vi "Write_Current_Row_to_log_file.vi"(0 "Current Time":dbl, 1 "Channel Names":string[](array[string]), 2 "Channel Values":string[](array[string]), 3 "Comments":string[](array[string]), 4 "User added comment":string) -> (7 "File Updated?":bool)   [LabVIEW 2020]
uses:
  ADAM_Global.vi
  Anemometry/Anemometry Sub Vis/Globals/Preference_global.vi
  Anemometry/Anemometry Sub Vis/Globals/Constants_global.vi
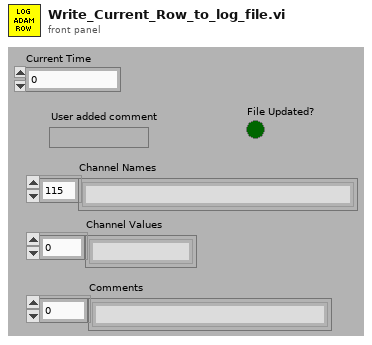
[diagram p1: front panel]
types:
  T1 = typedef "LVDateTimeRec.ctl" = cluster{"fractional second":dbl, "second":i32, "minute":i32, "hour":i32, "day of month":i32, "month":i32, "year":i32, "day of week":i32, "day of year":i32, "DST":i32}
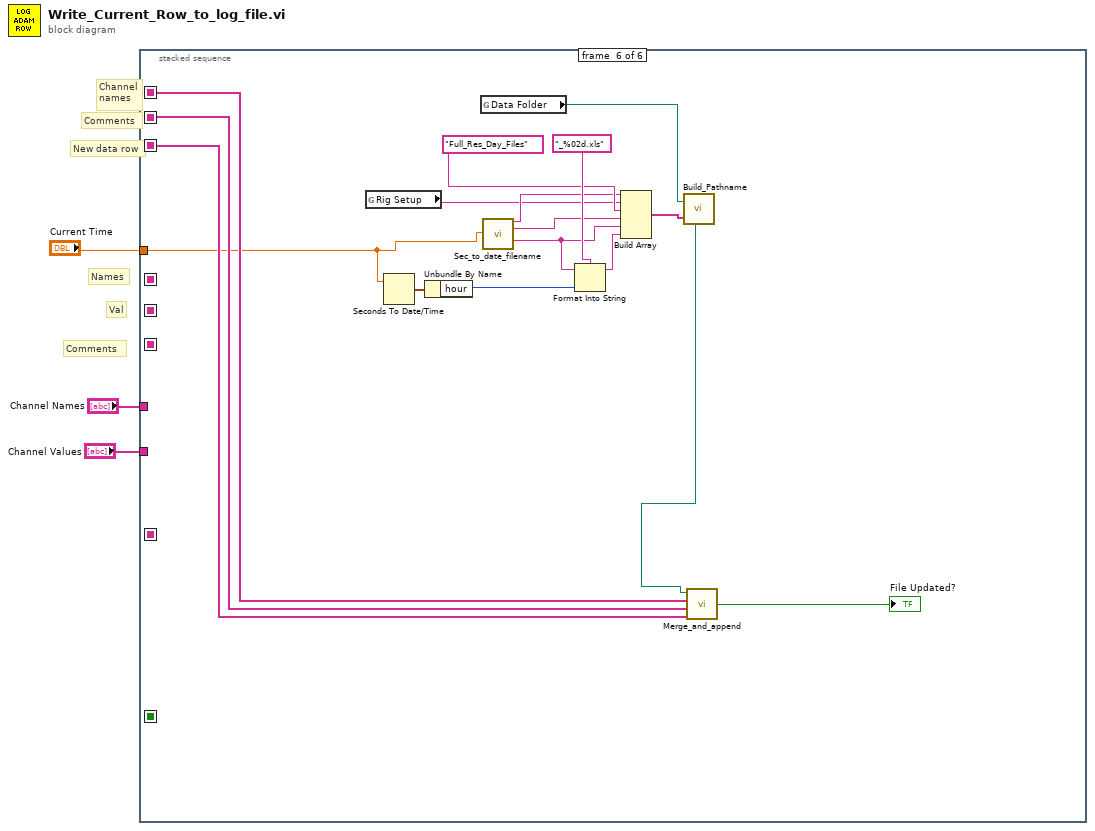
[diagram p0: block diagram]
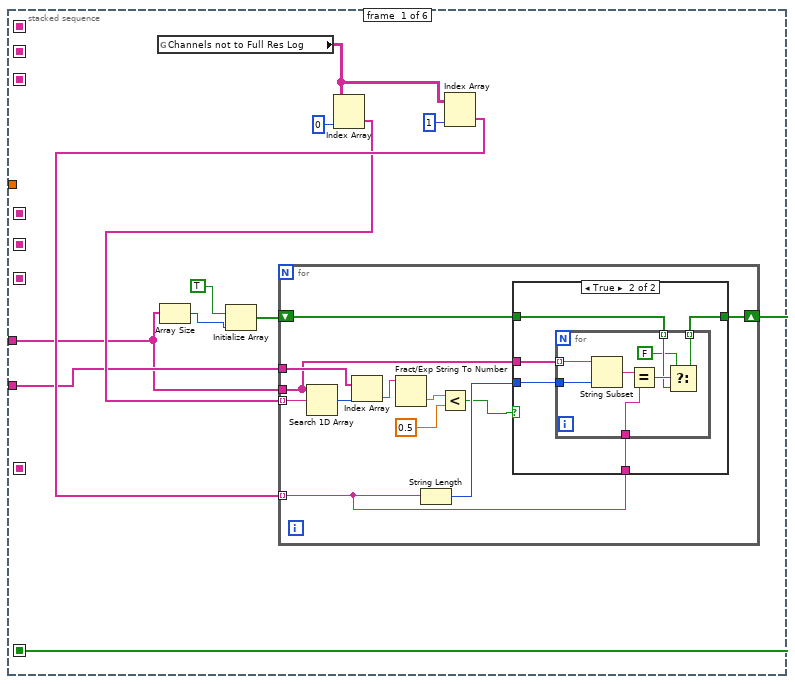
[diagram p2: hidden frame]
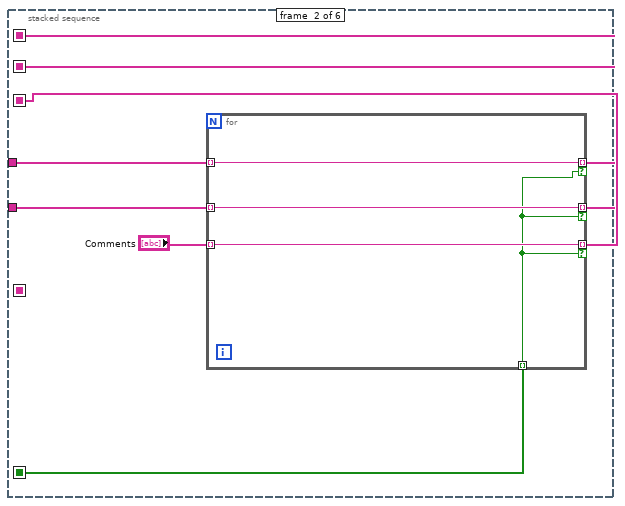
[diagram p4: hidden frame]
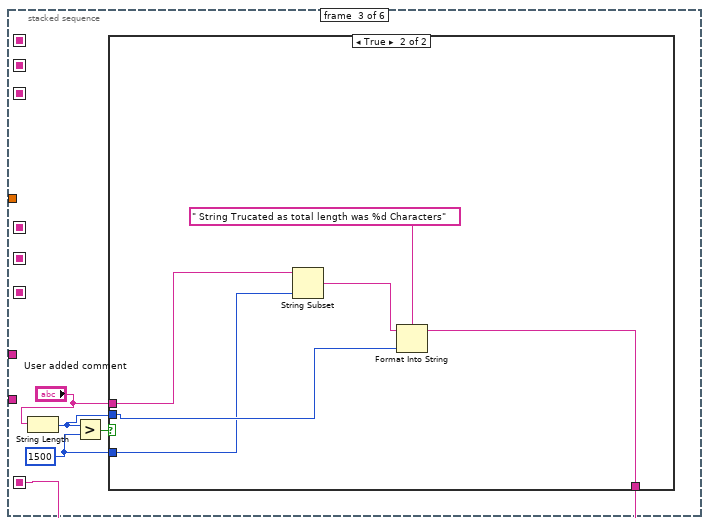
[diagram p5: hidden frame]
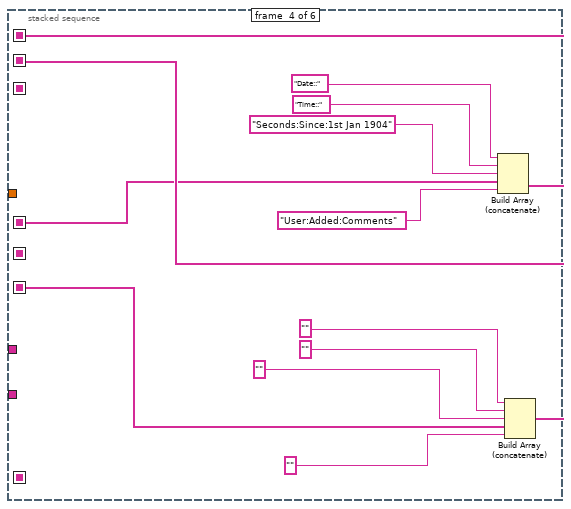
[diagram p7: hidden frame]
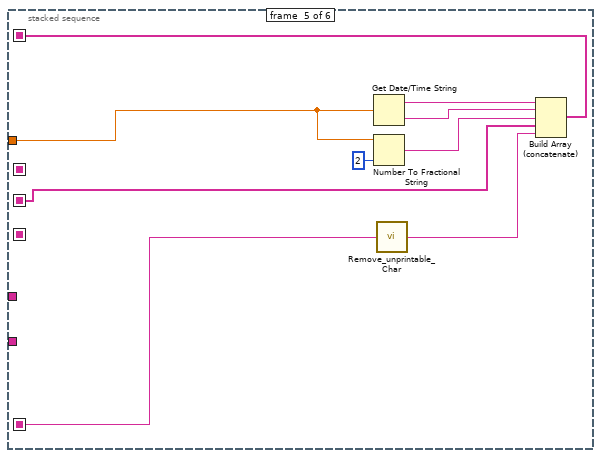
[diagram p8: hidden frame]
diagram:
  # "Comments"
  # "Names"
  # "Val"
  # "Comments"
  # "New data row"
  # "Channel\nnames"
  n1 = stacked-sequence {
    seq-local: [_ _ _ w72 _ _] -> [_ _ _ _ _ w101]
    seq-local: [_ _ _ _ w81 _] -> [_ _ _ _ _ w99]
    seq-local: [_ _ _ w66 _ _] -> [_ _ _ _ _ w100]
    seq-local: [_ _ w55 _ _ _] -> [_ _ _ _ w79 _]
    seq-local: [_ w45 _ _ _ _] -> [_ _ _ _ w78 _]
    seq-local: [_ w43 _ _ _ _] -> [_ _ _ w64 _ _]
    seq-local: [_ w47 _ _ _ _] -> [_ _ _ w65 _ _]
    seq-local: [w4 _ _ _ _ _] -> [_ w42 _ _ _ _]
    tunnel: "Current Time" -> [_ _ _ _ w76 w88]
    tunnel: "Channel Values" -> [w9 w44 _ _ _ _]
    tunnel: "Channel Names" -> [w5 w46 _ _ _ _]
    frame #0 {
      n2 = global read "ADAM_Global.vi" "Channels not to Full Res Log"() -> (w14:string[][])
      n3 = Array Size(array=w5) -> (size(s)=w7:i32)
      n4 = Initialize Array(TRUE, w7) -> (w8:bool[])
      n5 = Index Array(array=w14, index (col)=0 ("disabled index (col)")) -> (element=w10:string[])  [unwired: 1 in]
      n6 = Index Array(array=w14, index (col)=1 ("disabled index (col)")) -> (element=w11:string[])  [unwired: 1 in]
      n7 = for {
        tunnel: w11 -> [w19] mode=indexing
        tunnel: w5 -> [w17]
        tunnel: w10 -> [w26] mode=indexing
        tunnel: w9 -> [w24]
        shift-right: [w16] -> w4
        shift-left: w8 -> [w15]
        n8 = Search 1D Array(1D array=w17, element=w26) -> (index of element=w25:i32)  [unwired: 1 in]
        n9 = Index Array(array=w24, index=w25) -> (element=w23:string)
        n10 = Fract/Exp String To Number(string=w23) -> (number=w22:dbl)  [unwired: 3 in, 1 out]
        n11 = String Length(string=w19) -> (length=w20:i32)
        n12 = Less?(x=w22, y=0.5) -> (x < y?=w18:bool)
        n13 = case shown="True" w18 {
          tunnel: w17 -> [_ w32]
          tunnel: w20 -> [_ w31]
          tunnel: w19 -> [_ w30]
          tunnel: [w27 w28] -> w16
          tunnel: w15 -> [w27 w29]
          frame False {
          }
          frame True {
            n14 = for {
              tunnel: w32 -> [w37] mode=indexing
              tunnel: w31 -> [w39]
              tunnel: w30 -> [w38]
              tunnel: w29 -> [w35] mode=indexing
              tunnel: [w34] -> w28 mode=indexing
              n15 = String Subset(string=w37, length (rest)=w39) -> (substring=w40:string)  [unwired: 1 in]
              n16 = Equal?(x=w40, y=w38) -> (x = y?=w36:bool)
              n17 = Select(t=FALSE, s=w36, f=w35) -> (s? t:f=w34:bool)
            }
          }
        }
      }
    }
    frame #1 {
      n18 = for {
        tunnel: [w51] -> w47 mode=indexing if=w48
        tunnel: w46 -> [w51] mode=indexing
        tunnel: [w50] -> w45 mode=indexing if=w48
        tunnel: w44 -> [w50] mode=indexing
        tunnel: [w49] -> w43 mode=indexing if=w48
        tunnel: "Comments" -> [w49] mode=indexing
        tunnel: w42 -> [w48] mode=indexing
      }
    }
    frame #2 {
      w53 = 1500 ("y")
      n19 = String Length(string="User added comment") -> (length=w52:i32)
      n20 = Greater?(x=w52, y=w53) -> (0:w56:bool)
      n21 = case shown="True" w56 {
        tunnel: [w57 w58] -> w55
        tunnel: "User added comment" -> [w57 w63]
        tunnel: w53 -> [_ w59]
        tunnel: w52 -> [_ w62]
        frame False {
        }
        frame True {
          n22 = String Subset(string=w63, length (rest)=w59) -> (substring=w61:string)  [unwired: 1 out]
          n23 = Format Into String(format string=" String Trucated as total length was %d Characters", initial string=w61, w62) -> (resulting string=w58:string)  [unwired: 1 in, 1 out]
        }
      }
    }
    frame #3 {
      n24 = Build Array (concatenate)("Date::", "Time::", "Seconds:Since:1st Jan 1904", w65, "User:Added:Comments") -> (w72:string[])
      n25 = Build Array (concatenate)("", "", "", w64, "") -> (w66:string[])
    }
    frame #4 {
      n26 = Get Date/Time String(seconds (now)=w76) -> (date string=w84:string, time string=w83:string)  [unwired: 2 out]
      n27 = Number To Fractional String(number=w76, precision (6)=i16 2) -> (F-format string=w82:string)  [unwired: 2 in]
      n28 = call "Remove_unprintable_Char.vi"("Input String"=w79) -> ("Output String"=w80:string)
      n29 = Build Array (concatenate)(w84, w83, w82, w78, w80) -> (w81:string[])
    }
    frame #5 {
      n30 = global read "Preference_global.vi" "Rig Setup"() -> (w92:string)
      n31 = Seconds To Date/Time(time stamp (now)=w88) -> (date time rec=w93:T1)  [unwired: 1 in]
      n32 = Unbundle By Name(w93) -> ("hour"=w87:i32)
      n33 = global read "Constants_global.vi" "Data Folder"() -> (w91:path)
      n34 = call "Sec_to_date_filename.vi"("ss1904"=w88) -> ("YYYY"=w94:string, "mm-YYYY"=w86:string, "DD-mm-YYYY"=w85:string)  [unwired: 5 in, 7 out]
      n35 = Format Into String(format string="_%02d.xls", initial string=w85, w87) -> (resulting string=w97:string)  [unwired: 1 in, 1 out]
      n36 = Build Array(w94, w92, "Full_Res_Day_Files" ("Input Element"), w86, w85, w97) -> (w90:string[])
      n37 = call "Build_Pathname.vi"("PathElements"=w90, "PathnameIn"=w91) -> ("AppendedPath"=w89:path)
      n38 = call "Merge_and_append.vi"("New Row"=w99, "Comments"=w100, "Channel Names"=w101, "Path name"=w89) -> ("File Updated?"=→"File Updated?":bool)
    }
  }
